vi "Read_K2000_ValuesAveraged.vi"(8 "error in":errorcluster, 10 "No. Averaged Values":i32=10, 11 "VISA Refnum in":refnum<visa-resource-name>) -> (0 "error out":errorcluster, 2 "mean":dbl, 3 "VISA Refnum out":refnum<visa-resource-name>)   [LabVIEW 2021]
uses:
  <vilib>/Analysis/NI_AALBase.lvlib
panel:
  in  "y":dbl=0.1 format="%#_13g"
  out "Received":string
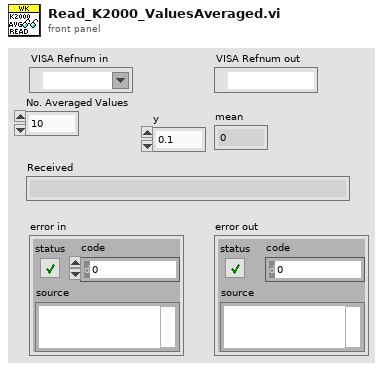
[diagram p1: front panel]
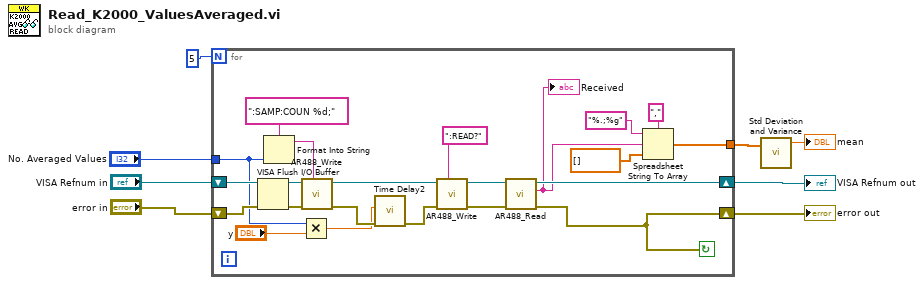
[diagram p0: block diagram]
diagram:
  n1 = for {
    N: 5 -> [_]
    tunnel: "No. Averaged Values" -> [w11]
    tunnel: [w23] -> w2
    shift-right: [w30] -> w8
    shift-left: "VISA Refnum in" -> [w27]
    shift-right: [w12] -> w7
    shift-left: "error in" -> [w24]
    stop <- w12 continue-if-true
    n2 = VISA Flush I/O Buffer(VISA resource name=w27, error in (no error)=w24) -> (VISA resource name out=w26:refnum<visa-resource-name>, error out=w25:errorcluster)  [unwired: 1 in]
    n3 = Format Into String(format string=":SAMP:COUN %d;" ("write"), w11) -> (resulting string=w28:string)  [unwired: 2 in, 1 out]
    n4 = Multiply(x=w11, y="y") -> (x*y=w9:dbl)
    n5 = call "AR488_Write.vi"("write"=w28, "error in (no error)"=w25, "VISA Refnum in"=w26) -> ("error out"=w14:errorcluster, "VISA Refnum out"=w18:refnum<visa-resource-name>)  [unwired: 7 in]
    n6 = call "Time Delay2"("error in (no error)"=w14, "Delay Time (s)"=w9) -> ("error out"=w13:errorcluster)  [unwired: 9 in]
    n7 = call "AR488_Write.vi"("write"=":READ?", "error in (no error)"=w13, "VISA Refnum in"=w18) -> ("error out"=w16:errorcluster, "VISA Refnum out"=w17:refnum<visa-resource-name>)  [unwired: 7 in]
    n8 = call "AR488_Read.vi"("error in"=w16, "VISA Refnum in"=w17) -> ("error out"=w12:errorcluster, "Received"=w21:string, "VISA Refnum out"=w30:refnum<visa-resource-name>)  [unwired: 6 in, 1 out]
    "Received" <- w21
    n9 = Spreadsheet String To Array(delimiter (Tab)=",", format string="%.;%g", spreadsheet string=w21, array type (2D Dbl)=dbl[] []) -> (array=w23:dbl[])
  }
  "VISA Refnum out" <- w8
  "error out" <- w7
  n10 = call <vilib>:"Std Deviation and Variance.vi"("X"=w2) -> ("mean"=→"mean":dbl)  [unwired: 1 in, 2 out]
